vi "SVL Integration (1 Ch).vi"(6 "reset filter (F)":bool, 7 "length units":i32(ring) items=["no change"=-1, "m"=0, "mm"=2, "microns"=3, "in"=1, "mils"=5], 8 "error in (no error)":errorcluster, 9 "highpass cutoff frequency  [Hz]":dbl=1.0 format="%.2f", 10 "integration type":T1(ring)=enum."double integration", 11 "scaled signal [EU]":waveform(dbl)={"t0"=timestamp(0 s since 1904-01-01), "dt"=1.0, "Y"=[0.0]}) -> (0 "error out":errorcluster, 2 "unit label":string, 3 "integrated signal":waveform(dbl)={"t0"=timestamp(0 s since 1904-01-01), "dt"=1.0, "Y"=[], "attributes"=variant("NI_SV_ChannelInfo"=variant(cluster{"sensor sensitivity [mV/EU]":dbl, "engineering units":enum16{"custom...", "V", "Pa", "g", "m/s^2", "m/s", "m", "in/s^2", "in/s", "in"}, "dB reference [EU]":dbl, "custom label":string, "weighting filter":enum16{"Linear", "A-weighting", "B-weighting", "C-weighting"}, "pregain [dB]":dbl} {"sensor sensitivity [mV/EU]"=1000.0, "engineering units"=enum."custom...", "dB reference [EU]"=1.0, "custom label"="not found*s^2", "weighting filter"=enum."Linear", "pregain [dB]"=0.0}))})   [LabVIEW 2017, in "SoundVib_Integration.lvlib"]
doc: "Converts acceleration to velocity or displacement using a time-domain waveform as the input. Wire data to the <B>scaled signal [EU]</B> input to determine the polymorphic instance to use or manually select the instance."
uses:
  <vilib>/addons/Sound and Vibration/svt_Integration/SoundVib_Integration.lvlib
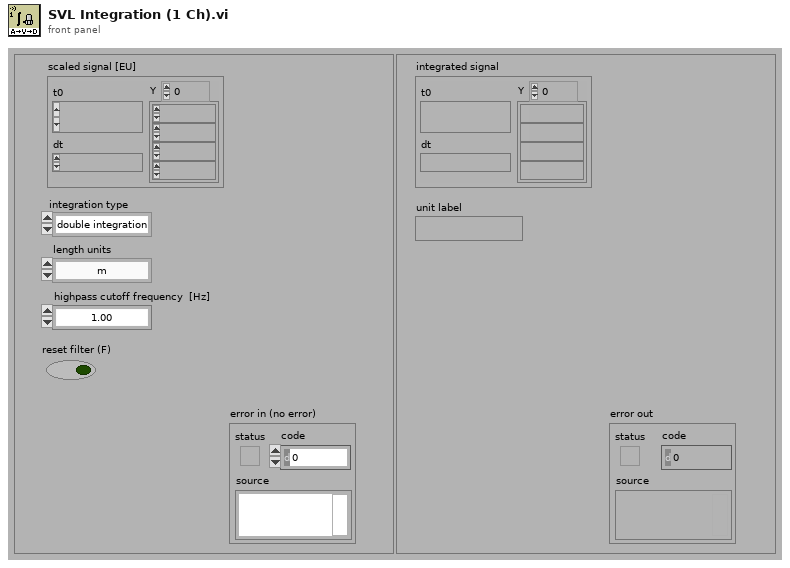
[diagram p1: front panel]
types:
  T1 = enum16{"single integration", "double integration"}
  T2 = cluster{"integration filter coefficients":cluster{"beta":dbl, "gamma":dbl, "alpha":dbl}, "highpass filter coefficients":cluster{"filter structure":enum32{"IIR 2nd Order", "IIR 4th Order"}, "Reverse Coefficients":dbl[], "Forward Coefficients":dbl[]}}
  T3 = cluster{"initial integration fiter state":cluster{"x(n-1) state":dbl, "y(n-1) state":dbl, "x(n-2) state":dbl, "y(n-2) state":dbl}, "initial highpass filter state":dbl[]}
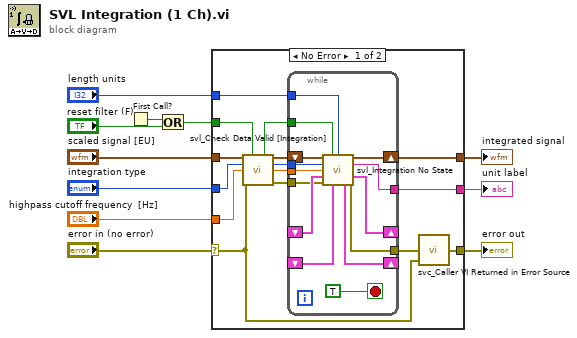
[diagram p0: block diagram]
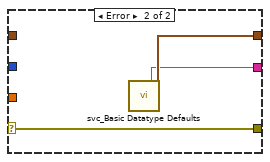
[diagram p2: hidden frame]
diagram:
  n1 = First Call?() -> (First Call?: T/F=w6:bool)
  n2 = Or(x=w6, y="reset filter (F)") -> (x .or. y?=w4:bool)
  n3 = case shown="No Error" "error in (no error)" {
    selector: "error in (no error)" -> [w12 w43]
    tunnel: "highpass cutoff frequency  [Hz]" -> [w19 _]
    tunnel: "scaled signal [EU]" -> [w21 _]
    tunnel: [w26 w42] -> w9
    tunnel: [w13 w43] -> w8
    tunnel: [w25 w41] -> w7
    tunnel: w4 -> [w23 _]
    tunnel: "integration type" -> [w20 _]
    tunnel: "length units" -> [w24 _]
    frame No Error {
      n4 = call <vilib>:"svl_Check Data Valid [Integration].vi"("signal in [X]"=w21, "reset (in)"=w23, "integration type"=w20, "highpass cutoff frequency"=w19, "error in (no error)"=w12) -> ("reset (out)"=w22:bool, "signal out [X]"=w15:waveform(dbl), "dup integration type"=w16:T1, "dup highpass cutoff frequency"=w17:dbl, "error out"=w18:errorcluster)  [unwired: 6 in]
      n5 = while {
        shift-left: _ -> [w34]
        shift-right: [w35] -> _
        shift-left: _ -> [w37]
        shift-right: [w36] -> _
        tunnel: w18 -> [w31]
        tunnel: w24 -> [w33]
        tunnel: w22 -> [w32]
        tunnel: [w38] -> w25
        tunnel: w17 -> [w30]
        tunnel: w16 -> [w29]
        tunnel: [w27] -> w14
        shift-right: [w39] -> w26
        shift-left: w15 -> [w28]
        stop <- TRUE stop-if-true
        n6 = call <vilib>:"svl_Integration No State.vi"("scaled signal [EU]"=w28, "reset filters"=w32, "length units"=w33, "integration type"=w29, "highpass cutoff frequency"=w30, "filter coefficents in"=w34, "error in (no error)"=w31, "initial filter state"=w37) -> ("scaled signal [EU]"=w39:waveform(dbl), "unit label"=w38:string, "filter coefficients out"=w35:T2, "final filter state"=w36:T3, "error out"=w27:errorcluster)  [unwired: 3 in]
      }
      n7 = call <vilib>:"svc_Caller VI Returned in Error Source.vi"("warning input to caller"=w12, "error in (no error)"=w14) -> ("error out"=w13:errorcluster)  [unwired: 3 in]
    }
    frame Error {
      n8 = call <vilib>:"svc_Basic Datatype Defaults.vi"() -> ("empty string"=w41:string, "empty waveform"=w42:waveform(dbl))  [unwired: 7 in, 11 out]
    }
  }
  "integrated signal" <- w9
  "error out" <- w8
  "unit label" <- w7
